vi "load_from_binary_file.vi"(6 "byte order (0:big-endian, network order)":T1(ring)=enum."little-endian", 8 "error in (no error)":errorcluster, 10 "Path":path, 11 "Image in":refnum<class "Image.lvclass">) -> (0 "error out":errorcluster, 3 "Image out":refnum<class "Image.lvclass">)   [LabVIEW 2010, in "Image.lvclass"]
uses:
  Image.lvclass
  error_codes_ring.ctl
  ErrorController/ErrorController/class_data.vi
  ErrorController/ErrorController/ErrorController.lvclass
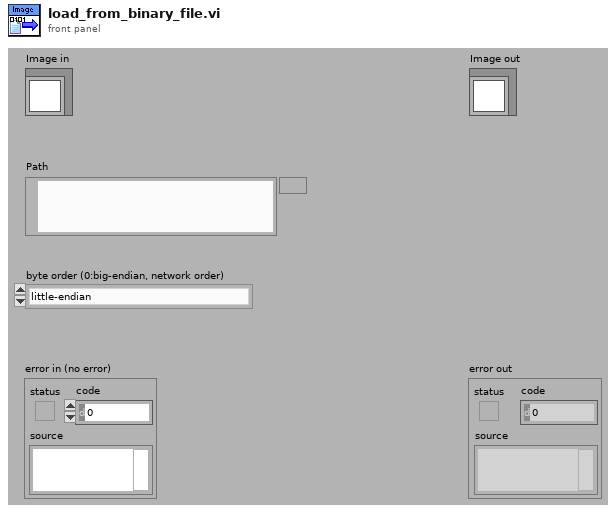
[diagram p1: front panel]
types:
  T1 = enum16{"big-endian, network order", "native, host order", "little-endian"}
  T2 = typedef "Color (U64)" = cluster{"Plane 3 (Blue)":u16, "Plane 2 (Green)":u16, "Plane 1 (Red)":u16, "Plane 4 (alpha)":u16}
  T3 = typedef "Image.lvclass/storage_mode.ctl" = enum16{"RAM", "disk"}
  T4 = typedef "Image Type" = u32
  T5 = typedef "IMAQ Image.ctl" = refnum<image>
  T6 = typedef "Image.lvclass/error_codes_ring.ctl" = u16
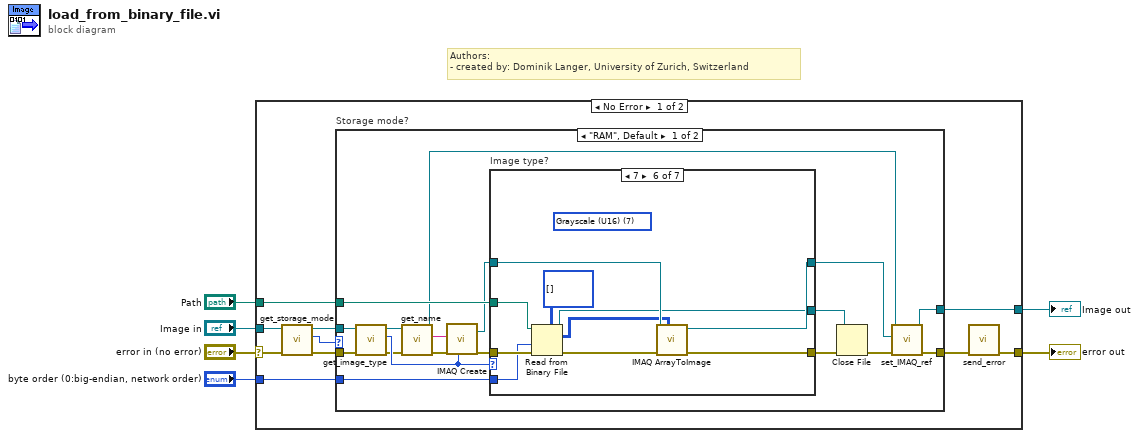
[diagram p0: block diagram]
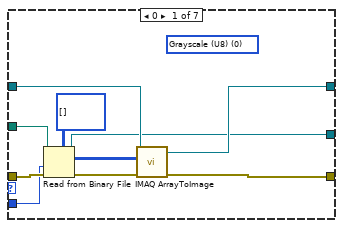
[diagram p2: hidden frame]
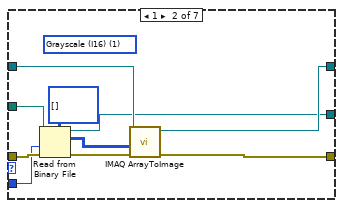
[diagram p3: hidden frame]
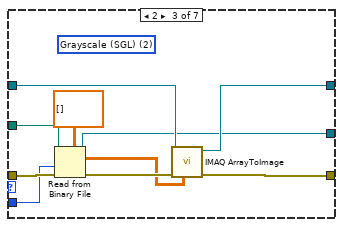
[diagram p4: hidden frame]
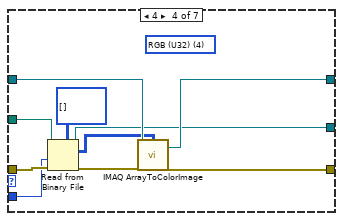
[diagram p5: hidden frame]
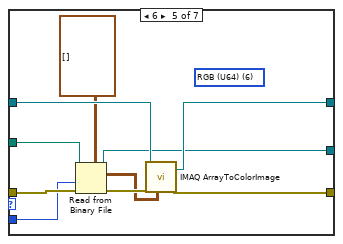
[diagram p6: hidden frame]
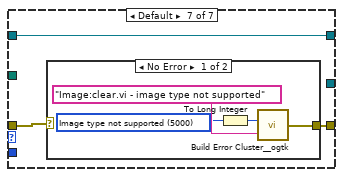
[diagram p7: hidden frame]
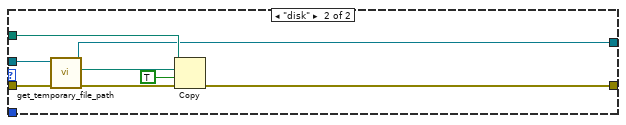
[diagram p9: hidden frame]
diagram:
  # "Authors: \n- created by: Dominik Langer, University of Zurich, Switzerland"
  n1 = case shown="No Error" "error in (no error)" {
    selector: "error in (no error)" -> [w14 w112]
    tunnel: [w8 w112] -> w5
    tunnel: [w15 w111] -> w3
    tunnel: "Image in" -> [w12 w111]
    tunnel: "Path" -> [w16 _]
    tunnel: "byte order (0:big-endian, network order)" -> [w9 _]
    frame No Error {
      n2 = call-dynamic "get_storage_mode.vi"("error in (no error)"=w14, "Image.lvclass in"=w12) -> ("error out"=w13:errorcluster, "storage mode"=w10:T3, "Image.lvclass out"=w11:refnum<class "Image.lvclass">)  [unwired: 7 out]
      n3 = case "Storage mode?" shown="\"RAM\", Default" w10 {
        tunnel: w16 -> [w34 w109]
        tunnel: [w33 w110] -> w7
        tunnel: [w32 w104] -> w15
        tunnel: w13 -> [w29 w108]
        tunnel: w11 -> [w28 w106]
        tunnel: w9 -> [w17 _]
        frame "RAM", Default {
          n4 = call-dynamic "get_image_type.vi"("error in (no error)"=w29, "Image.lvclass in"=w28) -> ("error out"=w25:errorcluster, "Image Type"=w26:T4, "Image.lvclass out"=w23:refnum<class "Image.lvclass">)  [unwired: 7 out]
          n5 = call-dynamic "get_name.vi"("error in (no error)"=w25, "Image in"=w23) -> ("error out"=w24:errorcluster, "name"=w21:string, "Image out"=w22:refnum<class "Image.lvclass">)  [unwired: 7 out]
          n6 = call "IMAQ Create"("Image Name"=w21, "Image Type"=w26, "error in (no error)"=w24) -> ("New Image"=w30:T5, "error out"=w27:errorcluster)  [unwired: 1 in, 1 out]
          n7 = case "Image type?" shown="7" w26 {
            tunnel: w30 -> [w39 w54 w58 w69 w80 w89 w97]
            tunnel: [w38 w53 w57 w68 w79 w90 w97] -> w31
            tunnel: w27 -> [w43 w51 w62 w73 w83 w92 w96]
            tunnel: [w42 w52 w61 w70 w82 w91 w95] -> w19
            tunnel: w34 -> [w37 w49 w60 w72 w81 w86 _]
            tunnel: [w36 w46 w56 w66 w76 w87 _] -> w18
            tunnel: w17 -> [w35 w45 w55 w65 w75 w85 _]
            frame 0 {
              (unwired) T4 0 items=["Grayscale (U8)", "Grayscale (I16)", "Grayscale (SGL)", "Complex (CSG)", "RGB (U32)", "HSL (U32)", "RGB (U64)", "Grayscale (U16)"] ("Image Type")
              n8 = Read from Binary File(5:u8[][] [], 8:w43, 9:w35, 11:w37) -> (0:w44:errorcluster, 2:w41:u8[][], 3:w36:refnum<file>)  [unwired: 1 in, 2 out]
              n9 = call "IMAQ ArrayToImage"("error in (no error)"=w44, "Image Pixels (U8)"=w41, "Image"=w39) -> ("error out"=w42:errorcluster, "Image Out"=w38:T5)  [unwired: 3 in, 4 out]
            }
            frame 1 {
              (unwired) T4 1 items=["Grayscale (U8)", "Grayscale (I16)", "Grayscale (SGL)", "Complex (CSG)", "RGB (U32)", "HSL (U32)", "RGB (U64)", "Grayscale (U16)"] ("Image Type")
              n10 = Read from Binary File(5:i16[][] [], 8:w51, 9:w45, 11:w49) -> (0:w50:errorcluster, 2:w47:i16[][], 3:w46:refnum<file>)  [unwired: 3 out]
              n11 = call "IMAQ ArrayToImage"("error in (no error)"=w50, "Image Pixels (I16)"=w47, "Image"=w54) -> ("error out"=w52:errorcluster, "Image Out"=w53:T5)  [unwired: 3 in, 4 out]
            }
            frame 2 {
              (unwired) T4 2 items=["Grayscale (U8)", "Grayscale (I16)", "Grayscale (SGL)", "Complex (CSG)", "RGB (U32)", "HSL (U32)", "RGB (U64)", "Grayscale (U16)"] ("Image Type")
              n12 = Read from Binary File(5:sgl[][] [], 8:w62, 9:w55, 11:w60) -> (0:w64:errorcluster, 2:w59:sgl[][], 3:w56:refnum<file>)  [unwired: 3 out]
              n13 = call "IMAQ ArrayToImage"("Image Pixels (Float)"=w59, "error in (no error)"=w64, "Image"=w58) -> ("error out"=w61:errorcluster, "Image Out"=w57:T5)  [unwired: 3 in, 4 out]
            }
            frame 4 {
              (unwired) T4 4 items=["Grayscale (U8)", "Grayscale (I16)", "Grayscale (SGL)", "Complex (CSG)", "RGB (U32)", "HSL (U32)", "RGB (U64)", "Grayscale (U16)"] ("Image Type")
              n14 = Read from Binary File(5:u32[][] [], 8:w73, 9:w65, 11:w72) -> (0:w71:errorcluster, 2:w67:u32[][], 3:w66:refnum<file>)  [unwired: 3 out]
              n15 = call "IMAQ ArrayToColorImage"("Image Pixels (U32)"=w67, "Image"=w69, "error in (no error)"=w71) -> ("Image Out"=w68:T5, "error out"=w70:errorcluster)  [unwired: 1 in, 1 out]
            }
            frame 6 {
              (unwired) T4 6 items=["Grayscale (U8)", "Grayscale (I16)", "Grayscale (SGL)", "Complex (CSG)", "RGB (U32)", "HSL (U32)", "RGB (U64)", "Grayscale (U16)"] ("Image Type")
              n16 = Read from Binary File(5:T2[][] [] ("Image Pixels (U64)"), 8:w83, 9:w75, 11:w81) -> (0:w84:errorcluster, 2:w77:T2[][], 3:w76:refnum<file>)  [unwired: 3 out]
              n17 = call "IMAQ ArrayToColorImage"("Image"=w80, "Image Pixels (U64)"=w77, "error in (no error)"=w84) -> ("Image Out"=w79:T5, "error out"=w82:errorcluster)  [unwired: 1 in, 1 out]
            }
            frame 7 {
              (unwired) T4 7 items=["Grayscale (U8)", "Grayscale (I16)", "Grayscale (SGL)", "Complex (CSG)", "RGB (U32)", "HSL (U32)", "RGB (U64)", "Grayscale (U16)"] ("Image Type")
              n18 = Read from Binary File(5:u16[][] [], 8:w92, 9:w85, 11:w86) -> (0:w93:errorcluster, 2:w88:u16[][], 3:w87:refnum<file>)  [unwired: 1 in, 2 out]
              n19 = call "IMAQ ArrayToImage"("Image Pixels (U16)"=w88, "error in (no error)"=w93, "Image"=w89) -> ("error out"=w91:errorcluster, "Image Out"=w90:T5)  [unwired: 3 in, 4 out]
            }
            frame Default {
              n20 = case shown="No Error" w96 {
                selector: w96 -> [_ w102]
                tunnel: [w101 w102] -> w95
                frame No Error {
                  w98 = T6 5000 items=["Image type not supported"=5000] ("Ring")
                  n21 = To Long Integer(number=w98) -> (32bit integer=w99:i32)
                  n22 = call <userlib>:"Build Error Cluster__ogtk.vi"("String to Prepend to source (\"\")"="Image:clear.vi - image type not supported" ("String to Prepend to source (\"\")"), "code"=w99) -> ("error out"=w101:errorcluster)
                }
                frame Error {
                }
              }
            }
          }
          n23 = Close File(refnum=w18, error in=w19) -> (error out=w20:errorcluster)  [unwired: 1 out]
          n24 = call-dynamic "set_IMAQ_ref.vi"("error in (no error)"=w20, "Image"=w31, "Image.lvclass in"=w22) -> ("error out"=w33:errorcluster, "Image.lvclass out"=w32:refnum<class "Image.lvclass">)  [unwired: 7 out]
        }
        frame "disk" {
          n25 = call-dynamic "get_temporary_file_path.vi"("error in (no error)"=w108, "Image.lvclass in"=w106) -> ("error out"=w107:errorcluster, "temporary file path"=w103:path, "Image.lvclass out"=w104:refnum<class "Image.lvclass">)  [unwired: 7 out]
          n26 = Copy(8:w107, 9:TRUE ("overwrite (F)"), 10:w103, 11:w109) -> (0:w110:errorcluster)  [unwired: 3 out]
        }
      }
      n27 = call "send_error.vi"("error in (no error)"=w7) -> ("error out"=w8:errorcluster)  [unwired: 10 in]
    }
    frame Error {
    }
  }
  "error out" <- w5
  "Image out" <- w3
